vi "IMAGE PATH CREATION PY.vi"(8 "error in (no error)":errorcluster, 11 "File Name :":string) -> (0 "error out":errorcluster, 2 "File Path":path, 3 "File Path String:":string)   [LabVIEW 2025]
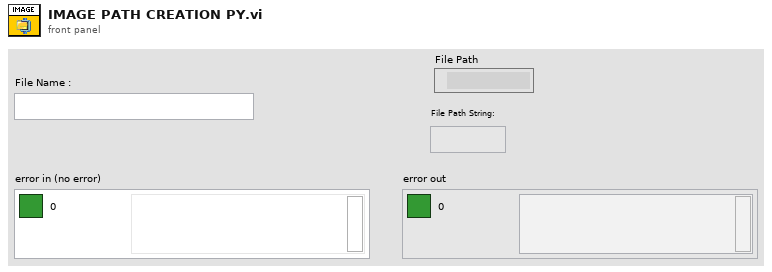
[diagram p1: front panel]
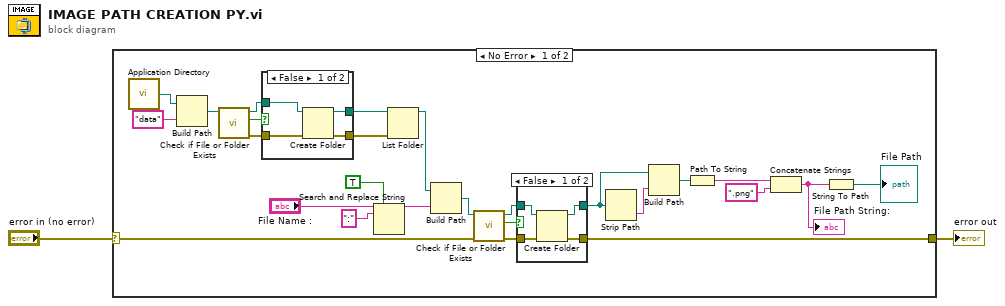
[diagram p0: block diagram]
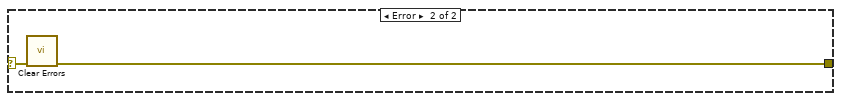
[diagram p4: hidden frame]
diagram:
  n1 = case shown="No Error" "error in (no error)" {
    selector: "error in (no error)" -> [w4 w42]
    tunnel: [w5 w41] -> w1
    frame No Error {
      n2 = call <vilib>:"Application Directory.vi"() -> ("Application Directory"=w21:path)
      n3 = Build Path(base path=w21, name or relative path="data") -> (appended path=w25:path)
      n4 = call <vilib>:"Check if File or Folder Exists.vi"("path"=w25) -> ("error out"=w22:errorcluster, "file or folder exists?"=w24:bool, "dup path"=w23:path)  [unwired: 8 in]
      n5 = case shown="False" w24 {
        tunnel: w23 -> [w38 w39]
        tunnel: w22 -> [w37 w40]
        tunnel: [w36 w40] -> w28
        tunnel: [w35 w39] -> w27
        frame False {
          n6 = Create Folder(path (use dialog)=w38, error in=w37) -> (created path=w35:path, error out=w36:errorcluster)  [unwired: 1 in, 1 out]
        }
        frame True {
        }
      }
      n7 = Search and Replace String(replace all?=TRUE ("replace all? (F)"), input string="File Name :", search string=":") -> (result string=w18:string)  [unwired: 5 in, 3 out]
      n8 = List Folder(path=w27, error in=w28) -> (path out=w16:path)  [unwired: 2 in, 3 out]
      n9 = Build Path(base path=w16, name or relative path=w18) -> (appended path=w17:path)
      n10 = call <vilib>:"Check if File or Folder Exists.vi"("error in (no error)"=w4, "path"=w17) -> ("error out"=w15:errorcluster, "file or folder exists?"=w13:bool, "dup path"=w14:path)  [unwired: 7 in]
      n11 = case shown="False" w13 {
        tunnel: w14 -> [w32 w33]
        tunnel: w15 -> [w31 w34]
        tunnel: [w30 w34] -> w5
        tunnel: [w29 w33] -> w8
        frame False {
          n12 = Create Folder(path (use dialog)=w32, error in=w31) -> (created path=w29:path, error out=w30:errorcluster)  [unwired: 1 in, 1 out]
        }
        frame True {
        }
      }
      n13 = Strip Path(path=w8) -> (name=w11:string)  [unwired: 1 out]
      n14 = Build Path(base path=w8, name or relative path=w11) -> (appended path=w12:path)
      n15 = Path To String(path=w12) -> (string=w9:string)
      n16 = Concatenate Strings(w9, ".png" ("string")) -> (w7:string)
      "File Path String:" <- w7
      n17 = String To Path(string=w7) -> (path=→"File Path":path)
    }
    frame Error {
      n18 = call <vilib>:"Clear Errors.vi"("error in (no error)"=w42) -> ("error out"=w41:errorcluster)  [unwired: 5 in, 1 out]
    }
  }
  "error out" <- w1
